vi "UI.Sequence.SelectCellOnDoubleClick.vi"(8 "error in (no error)":errorcluster, 9 "Coords":T4, 11 "State Variables":T1={"Aliases.All"=[], "Aliases.Outputs"=[], "UI.Sequence#ofColumns"=0, "SysDef.Path"=path "", "UI.SequenceRef"=refnum, "UI.StepInformationRef"=refnum, "UI.AbortRef"=refnum, "UI.GraphRef"=refnum, "UI.ViewRef"=refnum, "UI.IterationsRef"=refnum, "UI.IterationInformationRef"=refnum, "INI.Settings"={"Build Location"=path "C:/Simple Sequence Editor/SequenceRepo", "LoggingLocation"=path ""}, "NIVS.Workspace Event"=refnum, "UI.SkipChannel"=refnum, "NIVS.Launched?"=FALSE, "UI.DurationChannel"=refnum}) -> (0 "error out":errorcluster, 3 "State Variables out":T1={"Aliases.All"=[], "Aliases.Outputs"=[], "UI.Sequence#ofColumns"=0, "SysDef.Path"=path "", "UI.SequenceRef"=refnum, "UI.StepInformationRef"=refnum, "UI.AbortRef"=refnum, "UI.GraphRef"=refnum, "UI.ViewRef"=refnum, "UI.IterationsRef"=refnum, "UI.IterationInformationRef"=refnum, "INI.Settings"={"Build Location"=path "C:/Simple Sequence Editor/SequenceRepo", "LoggingLocation"=path ""}, "NIVS.Workspace Event"=refnum, "UI.SkipChannel"=refnum, "NIVS.Launched?"=FALSE, "UI.DurationChannel"=refnum})   [LabVIEW 2013, in "Simple Sequence Tools - Editor.lvlib"]
uses:
  Simple Sequence Tools - Editor.lvlib
  Types/Main.StateVariables.ctl
  Shared/Types/Channel.Properties.ctl
  Shared/Types/INI.Settings
  <vilib>/Utility/miscctls.llb/LVPoint32TypeDef.ctl
  Shared/SubVIs/Main.Constants.vi
  Shared/Simple Sequence Tools - Shared.lvlib
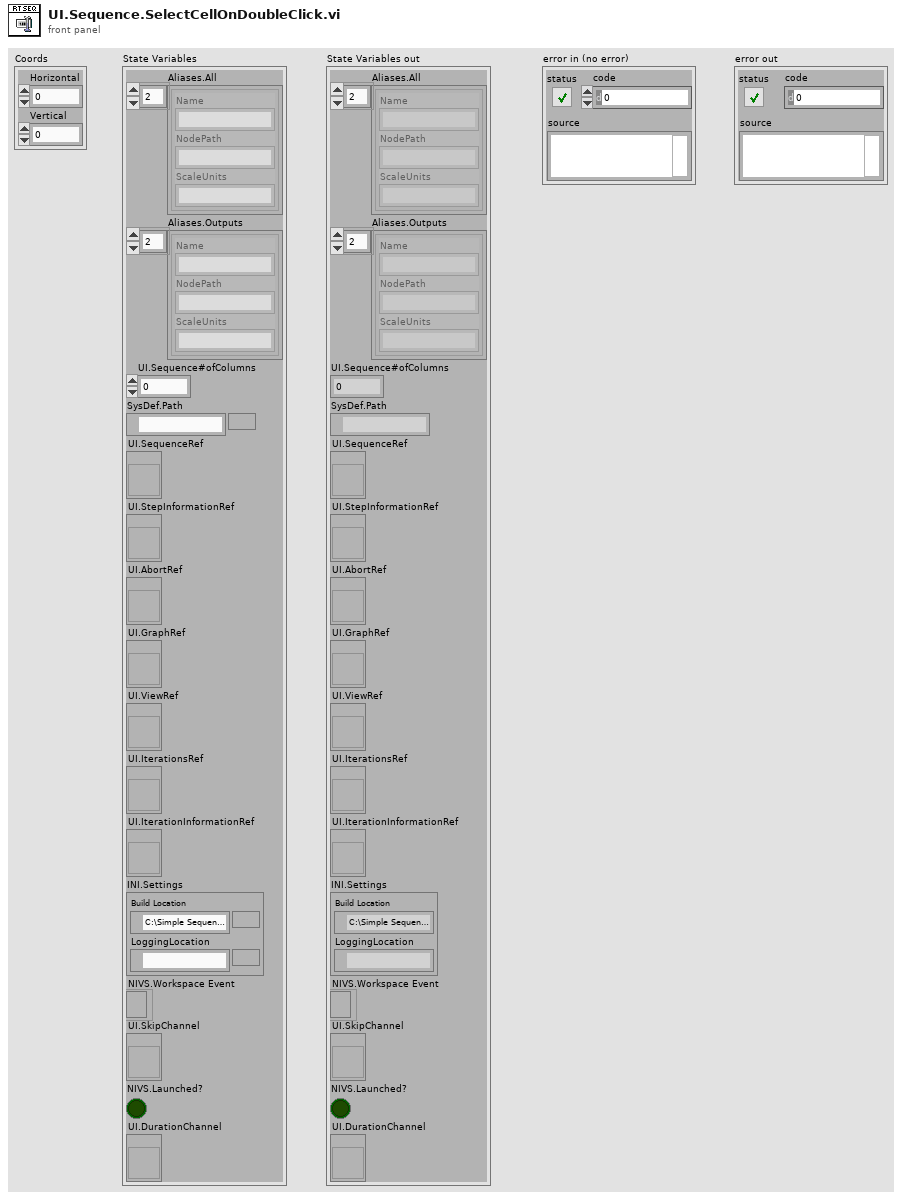
[diagram p1: front panel]
types:
  T1 = typedef "Simple Sequence Tools - Editor.lvlib/Main.StateVariables.ctl" = cluster{"Aliases.All":T2[], "Aliases.Outputs":T2[], "UI.Sequence#ofColumns":i32, "SysDef.Path":path, "UI.SequenceRef":refnum<vi>, "UI.StepInformationRef":refnum<vi>, "UI.AbortRef":refnum<vi>, "UI.GraphRef":refnum<vi>, "UI.ViewRef":refnum<vi>, "UI.IterationsRef":refnum<vi>, "UI.IterationInformationRef":refnum<vi>, "INI.Settings":T3, "NIVS.Workspace Event":refnum<event-registration>, "UI.SkipChannel":refnum<vi>, "NIVS.Launched?":bool, "UI.DurationChannel":refnum<vi>}
  T2 = typedef "Simple Sequence Tools - Shared.lvlib/Channel.Properties.ctl" = cluster{"Name":string, "NodePath":string, "ScaleUnits":string}
  T3 = typedef "Simple Sequence Tools - Shared.lvlib/INI.Settings" = cluster{"Build Location":path, "LoggingLocation":path}
  T4 = typedef "LVPoint32TypeDef.ctl" = cluster{"Horizontal":i32, "Vertical":i32}
  T5 = typedef "LVRowAndColumnTypeDef.ctl" = cluster{"Row":i32, "Column":i32}
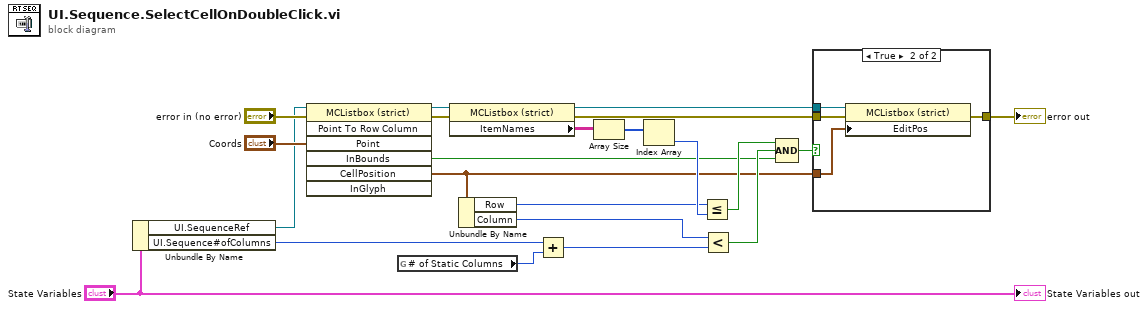
[diagram p0: block diagram]
diagram:
  n1 = Unbundle By Name("State Variables") -> ("UI.SequenceRef"=w1:refnum<vi>, "UI.Sequence#ofColumns"=w18:i32)
  n2 = invoke class="MCListbox (strict)" method="Point To Row Column"(reference=w1, error in="error in (no error)", "Point"="Coords") -> (reference out=w3:refnum<vi>, error out=w8:errorcluster, "InBounds"=w2:bool, "CellPosition"=w12:T5)  [unwired: 4 in, 3 out]
  n3 = global read "Main.Constants.vi" "# of Static Columns"() -> (w19:u32)
  n4 = property class="MCListbox (strict)"(reference=w3, error in=w8) -> (reference out=w7:refnum<vi>, error out=w9:errorcluster, "ItemNames"=w10:string[][])
  n5 = Unbundle By Name(w12) -> ("Row"=w13:i32, "Column"=w20:i32)
  n6 = Add(x=w18, y=w19) -> (x+y=w21:u32)
  n7 = Array Size(array=w10) -> (size(s)=w11:i32[])
  n8 = Index Array(array=w11) -> (element=w14:i32)  [unwired: 1 in]
  n9 = Less Or Equal?(x=w13, y=w14) -> (x <= y?=w16:bool)
  n10 = Less?(x=w20, y=w21) -> (x < y?=w22:bool)
  n11 = Compound Arithmetic op=AND(w16, w22, w2) -> (w15:bool)
  n12 = case shown="True" w15 {
    tunnel: w7 -> [_ w27]
    tunnel: w12 -> [_ w26]
    tunnel: w9 -> [w23 w25]
    tunnel: [w23 w24] -> w6
    frame False {
    }
    frame True {
      n13 = property class="MCListbox (strict)"(reference=w27, error in=w25, "EditPos"=w26) -> (error out=w24:errorcluster)  [unwired: 1 out]
    }
  }
  "error out" <- w6
  "State Variables out" <- "State Variables"
